vi "cRIO - FTP Module.vi"(5 "List":bool, 6 "Destination Folder (on local host)":path=path "C:/Temp/cRIO copied raw Data", 7 "Copy":bool, 8 "Error In":errorcluster, 9 "Source File Path (on RT Target)":string="c:\\ni-rt\\LabVIEW Data\\SRTRS4070\\Data\\2014\\04\\0090300849_20140402_130159.dat", 10 "Source Folder (on RT target)":string="c:\\ni-rt\\LabVIEW Data\\SRTRS4070\\Data\\2014\\04\\", 11 "IP address of remote RT target":string="192.168.1.50") -> (0 "Error Out":errorcluster, 2 "File Specification":T1={"Remote Path"="c:\\ni-rt\\LabVIEW Data\\SRTRS4070\\Data\\2014\\04\\0090300849_20140402_130159.dat", "Local Path"=path "C:/Temp/cRIO copied Data/0090300849_20140402_130159.dat", "Binary"=FALSE}, 3 "Files in cRIO":string[](array[string])=["c:\\ni-rt\\LabVIEW Data\\SRTRS4070\\Data\\2014\\04\\0090300849_20140402_130159.dat", "c:\\ni-rt\\LabVIEW Data\\SRTRS4070\\Data\\2014\\04\\0090300849_20140402_130231.dat", "c:\\ni-rt\\LabVIEW Data\\SRTRS4070\\Data\\2014\\04\\0090300850_20140402_130537.dat", "c:\\ni-rt\\LabVIEW Data\\SRTRS4070\\Data\\2014\\04\\0090300850_20140402_130730.dat", "c:\\ni-rt\\LabVIEW Data\\SRTRS4070\\Data\\2014\\04\\0090300693_20140402_131057.dat", "c:\\ni-rt\\LabVIEW Data\\SRTRS4070\\Data\\2014\\04\\0090300694_20140402_131444.dat", "c:\\ni-rt\\LabVIEW Data\\SRTRS4070\\Data\\2014\\04\\0090300852_20140402_131856.dat", "c:\\ni-rt\\LabVIEW Data\\SRTRS4070\\Data\\2014\\04\\0090300853_20140402_131954.dat", "c:\\ni-rt\\LabVIEW Data\\SRTRS4070\\Data\\2014\\04\\0090300853_20140402_132648.dat", "c:\\ni-rt\\LabVIEW Data\\SRTRS4070\\Data\\2014\\04\\0090300853_20140402_132811.dat"], 4 "Destination File Path (on local host)":path)   [LabVIEW 2013]
uses:
  <vilib>/FTP/NI_FTP.lvlib
panel:
  in  "local port":u16
  in  "timeout ms (60000)":i32=10000
  in  "remote port (21)":u16=21
  # "ftp://192.168.1.50/ni-rt/LabVIEW%20Data/SRTRS4070/Data/2014/04/"
  # "c:\\ni-rt.ini"
  # "u:\\"
  # "Remote Path"
  # "To get USB drive"
  # "c:\\ni-rt\\LabVIEW Data\\SRTRS4070\\Data\\2014\\04\\0090300849_20140402_130159.dat"
  # "Local Path"
  # "C:\\Temp\\cRIO copied Data\\0090300849_20140402_130159.dat"
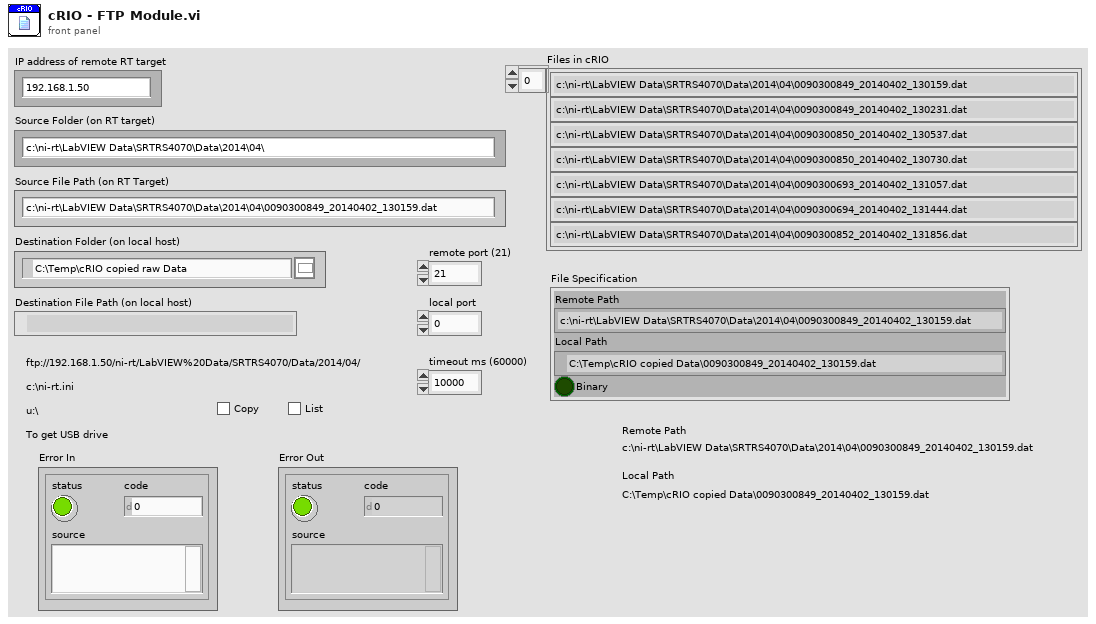
[diagram p1: front panel]
types:
  T1 = cluster{"Remote Path":string, "Local Path":path, "Binary":bool}
  T2 = cluster{"remote file path":string, "local file path":path, "binary":bool}
  T3 = typedef "NI_FTP.lvlib/FTP Session.ctl" = refnum<k5>
  T4 = typedef "NI_FTP.lvlib/FTP File Info.ctl" = cluster{"type":enum16{"unknown", "file", "dir", "link"}, "permissions":string, "owner":string, "group":string, "size":i32, "date":string, "name":string, "link name":string}
  T5 = cluster{"remote file path":string, "local file path":path, "binary":bool}[]
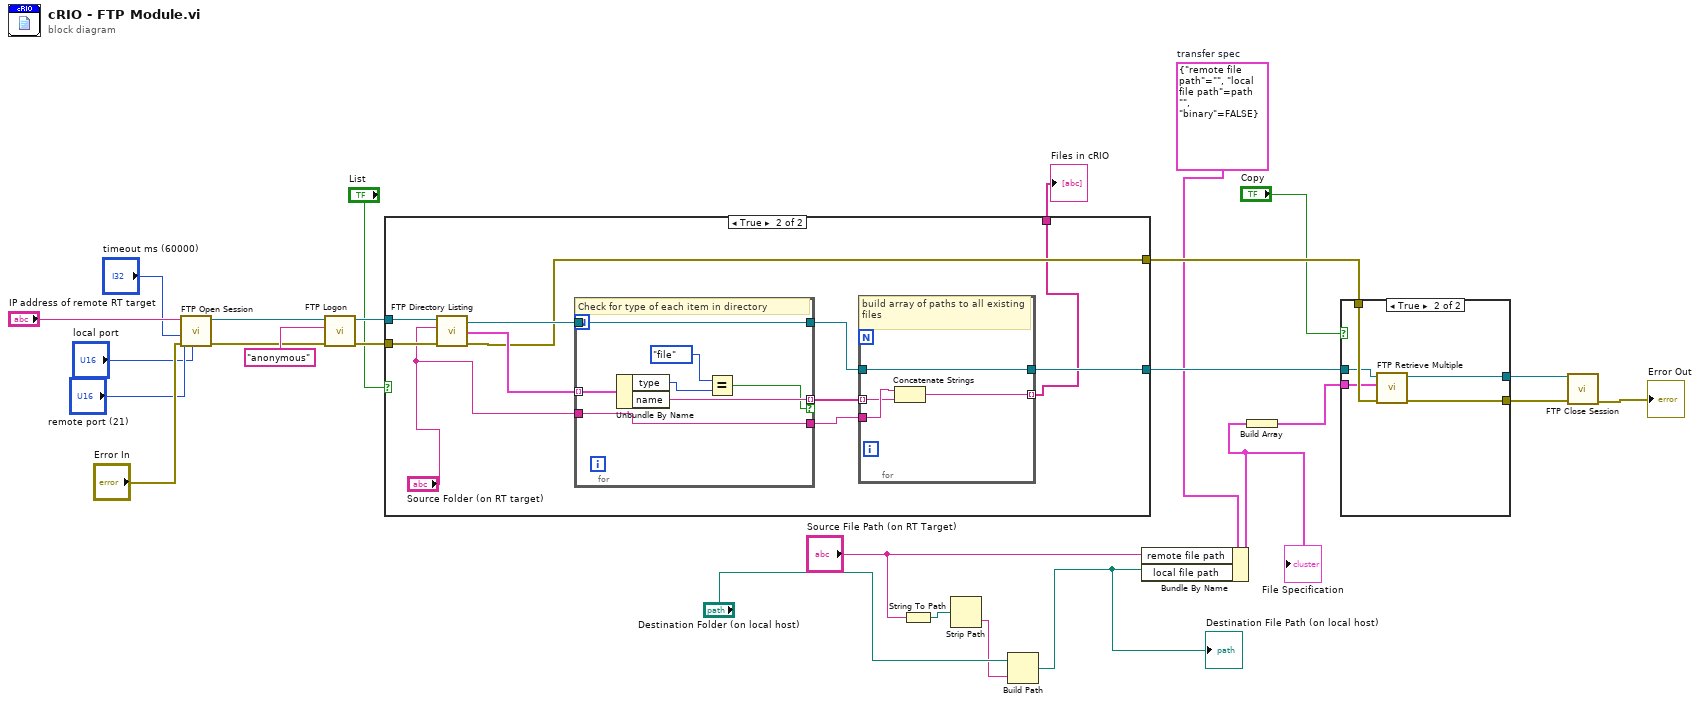
[diagram p0: block diagram]
diagram:
  w11 = T2 {"remote file path"="", "local file path"=path "", "binary"=FALSE}  # transfer spec
  n1 = call <vilib>:"FTP Open Session.vi"("local port"="local port", "error in (no error)"="Error In", "timeout ms (60000)"="timeout ms (60000)", "remote port (21)"="remote port (21)", "address"="IP address of remote RT target") -> ("error out"=w20:errorcluster, "ftp session"=w26:T3)  [unwired: 3 in, 2 out]
  n2 = call <vilib>:"FTP Logon.vi"("error in (no error)"=w20, "user"="anonymous", "ftp session"=w26) -> ("error out"=w19:errorcluster, "ftp session out"=w25:T3)  [unwired: 5 in, 2 out]
  n3 = case shown="True" "List" {
    tunnel: w25 -> [w27 w39]
    tunnel: w19 -> [w28 w36]
    tunnel: [w28 w35] -> w18
    tunnel: [w27 w31] -> w14
    tunnel: [_ w29] -> w4
    frame False {
    }
    frame True {
      n4 = call <vilib>:"FTP Directory Listing.vi"("error in (no error)"=w36, "directory path"="Source Folder (on RT target)", "ftp session"=w39) -> ("error out"=w35:errorcluster, "ftp session out"=w37:T3, "dir list"=w38:T4[])  [unwired: 4 in, 2 out]
      n5 = for {
        tunnel: w38 -> [w50] mode=indexing
        tunnel: [w49] -> w32
        tunnel: w37 -> [w49]
        tunnel: [w46] -> w34 mode=indexing if=w45
        tunnel: [w44] -> w33
        tunnel: "Source Folder (on RT target)" -> [w44]
        # "Check for type of each item in directory"
        n6 = Unbundle By Name(w50) -> ("type"=w48:enum16{"unknown", "file", "dir", "link"}, "name"=w46:string)
        n7 = Equal?(x=enum16{"unknown", "file", "dir", "link"}."file", y=w48) -> (x = y?=w45:bool)
      }
      n8 = for {
        tunnel: w34 -> [w40] mode=indexing
        tunnel: w33 -> [w41]
        tunnel: [w43] -> w29 mode=indexing
        tunnel: [w42] -> w31
        tunnel: w32 -> [w42]
        # "build array of paths to all existing files"
        n9 = Concatenate Strings(w41, w40) -> (w43:string)
      }
    }
  }
  "Files in cRIO" <- w4
  n10 = String To Path(string="Source File Path (on RT Target)") -> (path=w8:path)
  n11 = Strip Path(path=w8) -> (name=w6:string)  [unwired: 1 out]
  n12 = Build Path(base path="Destination Folder (on local host)", name or relative path=w6) -> (appended path=w5:path)
  "Destination File Path (on local host)" <- w5
  n13 = Bundle By Name(cluster=w11, "remote file path"="Source File Path (on RT Target)", "local file path"=w5) -> (w10:T2)
  "File Specification" <- w10
  n14 = Build Array(w10) -> (w13:T5)
  n15 = case shown="True" "Copy" {
    tunnel: [w52 w57] -> w22
    tunnel: [w51 w56] -> w21
    tunnel: w18 -> [w51 w55]
    tunnel: w13 -> [_ w54]
    tunnel: w14 -> [w52 w53]
    frame False {
    }
    frame True {
      n16 = call <vilib>:"FTP Retrieve Multiple.vi"("error in (no error)"=w55, "file specifications"=w54, "ftp session"=w53) -> ("error out"=w56:errorcluster, "ftp session out"=w57:T3)  [unwired: 5 in, 2 out]
    }
  }
  n17 = call <vilib>:"FTP Close Session.vi"("error in (no error)"=w21, "ftp session"=w22) -> ("error out"=→"Error Out":errorcluster)  [unwired: 6 in, 3 out]
